vi "Run.vi"(8 "error in (no error)":errorcluster caption="entrée d'erreur (pas d'erreur)", 11 "Regression.lvclass":refnum<class "Regression.lvclass">) -> (0 "error out":errorcluster caption="sortie d'erreur", 2 "Data":T1, 3 "Regression.lvclass":refnum<class "Regression.lvclass">)   [LabVIEW 2020, in "Regression.lvclass"]
doc: "Returns :\n\nX : array of shape [n_samples, n_features]\nThe input samples.\n\ny : array of shape [n_samples] or [n_samples, n_targets]\nThe output values.\n\ncoef : array of shape [n_features] or [n_features, n_targets], optional\nThe coefficient of the underlying linear model. It is returned only if coef is True."
uses:
  Regression.lvclass
  Regression.lvclass/Regression.ctl
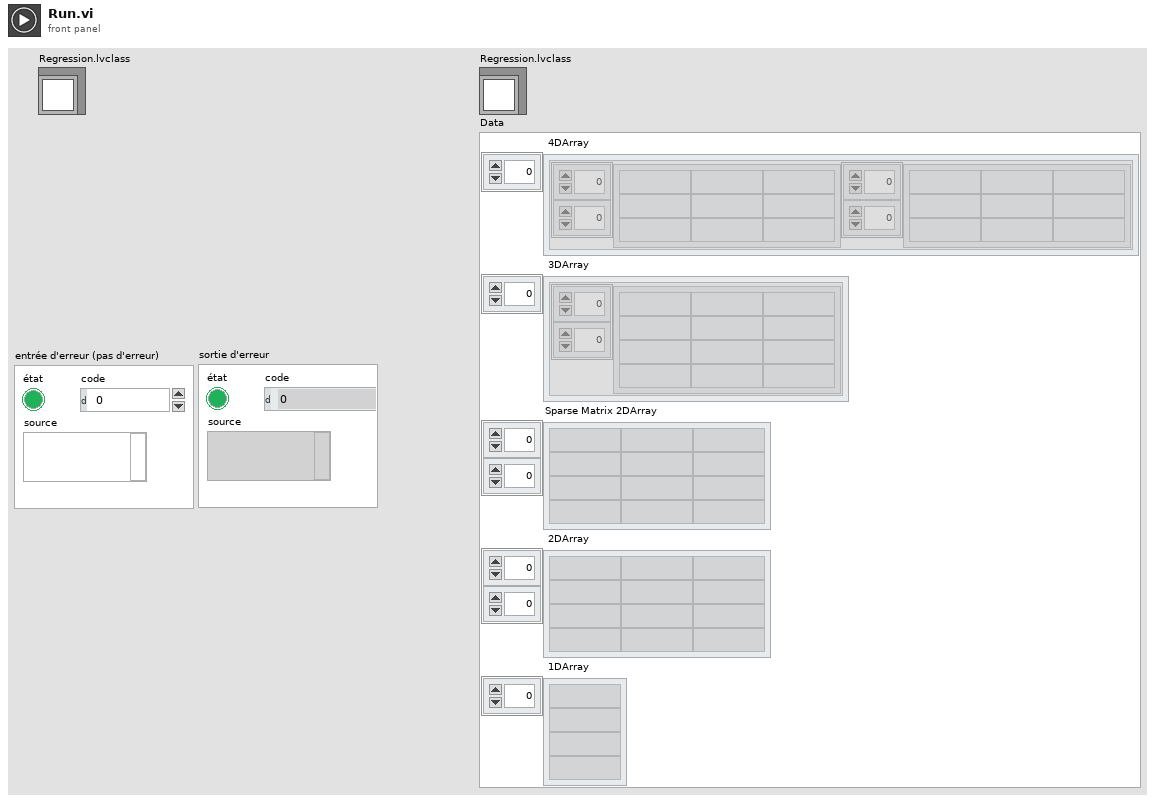
[diagram p1: front panel]
types:
  T1 = cluster{" 4DArray":cluster{"1":string[][], "2":string[][]}[], " 3DArray":cluster{"Tableau":string[][]}[], "Sparse Matrix 2DArray":string[][], " 2DArray":string[][], " 1DArray":string[]}
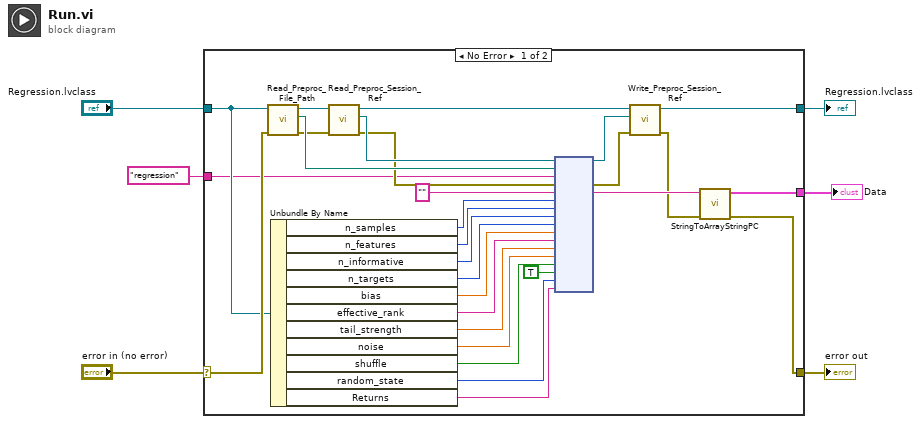
[diagram p0: block diagram]
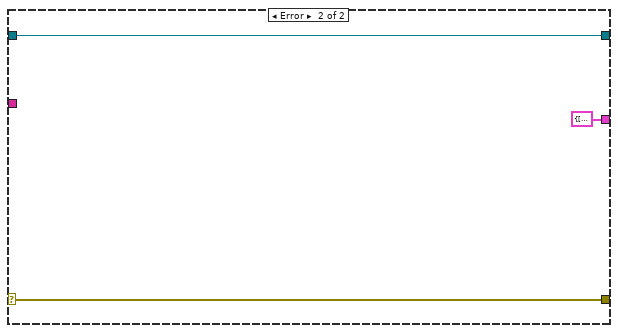
[diagram p2: hidden frame]
diagram:
  n1 = case shown="No Error" "error in (no error)" {
    selector: "error in (no error)" -> [w24 w38]
    tunnel: [w8 w38] -> w5
    tunnel: [w11 w37] -> w3
    tunnel: "Regression.lvclass" -> [w23 w37]
    tunnel: "regression" -> [w22 _]
    tunnel: [w7 T1 {" 4DArray"=[], " 3DArray"=[], "Sparse Matrix 2DArray"=[], " 2DArray"=[], " 1DArray"=[]} ("Data")] -> w1
    frame No Error {
      n2 = call-dynamic "Read_Preproc_File_Path.vi"("error in (no error)"=w24, "Python in"=w23) -> ("error out"=w30:errorcluster, "File_Path"=w33:path, "Python out"=w35:refnum<class "Regression.lvclass">)  [unwired: 7 in]
      n3 = Unbundle By Name(w23) -> ("n_samples"=w26:u32, "n_features"=w25:u32, "n_informative"=w21:u32, "n_targets"=w20:u32, "bias"=w19:dbl, "effective_rank"=w18:string, "tail_strength"=w17:dbl, "noise"=w16:dbl, "shuffle"=w15:bool, "random_state"=w13:i32, "Returns"=w12:string)
      n4 = call-dynamic "Read_Preproc_Session_Ref.vi"("error in (no error)"=w30, "Python in"=w35) -> ("error out"=w31:errorcluster, "Session_ref"=w32:refnum<k35>, "Python out"=w34:refnum<class "Regression.lvclass">)  [unwired: 7 in]
      n5 = node(w32, w33, w22, w31, "", w26, w25, w21, w20, w19, w18, w17, w16, w15, TRUE, w13, w12) -> (w27:refnum<k35>, w29:errorcluster, w10:string)  [unwired: 12 in, 2 out]
      n6 = call-dynamic "Write_Preproc_Session_Ref.vi"("error in (no error)"=w29, "Session_ref"=w27, "Python in"=w34) -> ("error out"=w9:errorcluster, "Python out"=w11:refnum<class "Regression.lvclass">)  [unwired: 7 in]
      n7 = call "StringToArrayStringPC.vi"("sortie d'erreur"=w9, "Return value"=w10) -> ("sortie d'erreur"=w8:errorcluster, "Data"=w7:T1)  [unwired: 8 in]
    }
    frame Error {
    }
  }
  "error out" <- w5
  "Regression.lvclass" <- w3
  "Data" <- w1
